vi "8_16byte.vi"() -> ()   [LabVIEW 2020]
panel:
  out "array":u8[][](array[numeric]) format="%.0x"
  out "number":u8[](array[numeric]) format="%.0x"
  out "Array":string[](array[string])
  out "text":string
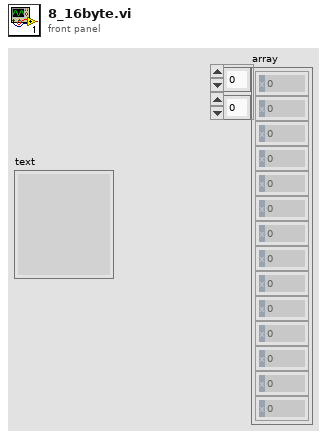
[diagram p1: front panel]
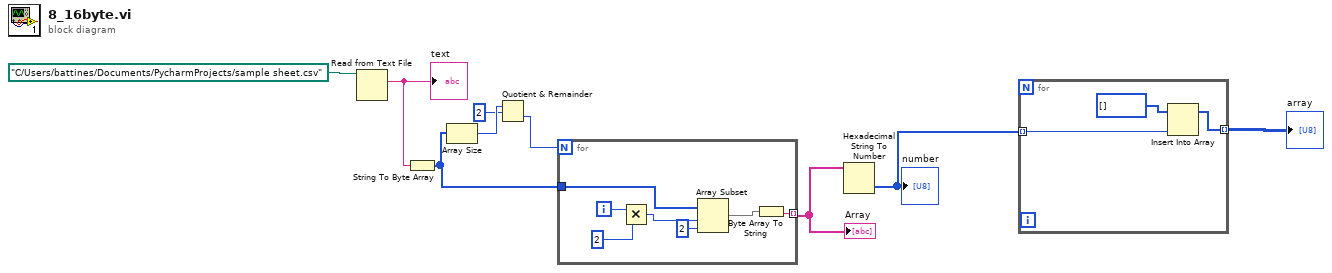
[diagram p0: block diagram]
diagram:
  n1 = Read from Text File(file (use dialog)=path "C:/Users/battines/Documents/PycharmProjects/sample sheet.csv") -> (text=w8:string)  [unwired: 3 in, 3 out]
  "text" <- w8
  n2 = String To Byte Array(string=w8) -> (unsigned byte array=w5:u8[])
  n3 = Array Size(array=w5) -> (size(s)=w7:i32)
  n4 = Quotient & Remainder(x=w7, y=2) -> (floor(x/y)=w4:i32)  [unwired: 1 out]
  n5 = for {
    N: w4 -> [_]
    tunnel: w5 -> [w16]
    tunnel: [w11] -> w3 mode=indexing
    i -> [w15]
    n6 = Multiply(x=w15, y=2) -> (x*y=w13:i32)
    n7 = Array Subset(array=w16, index=w13, length=2) -> (w12:u8[])
    n8 = Byte Array To String(unsigned byte array=w12) -> (string=w11:string)
  }
  "Array" <- w3
  n9 = Hexadecimal String To Number(string=w3) -> (number=w2:u32[])  [unwired: 2 in, 1 out]
  "number" <- w2
  n10 = for {
    tunnel: [w19] -> w1 mode=indexing
    tunnel: w2 -> [w17] mode=indexing
    n11 = Insert Into Array(array=u8[] [], new element=w17) -> (w19:u8[])  [unwired: 1 in]
  }
  "array" <- w1
